vi "UI.vi"() -> ()   [LabVIEW 2020]
panel:
  out "elements":dbl[](array[numeric])
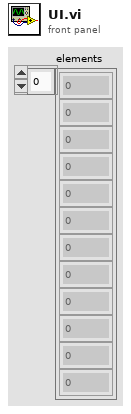
[diagram p1: front panel]
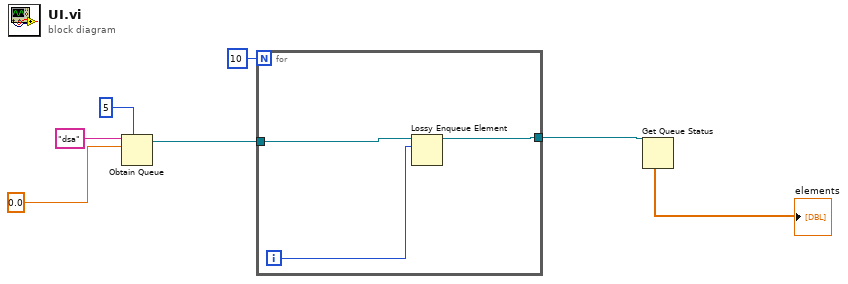
[diagram p0: block diagram]
diagram:
  n1 = Obtain Queue(max queue size (-1, unlimited)=5, name (unnamed)="dsa", element data type=0.0) -> (queue out=w3:refnum<queue>)  [unwired: 2 in, 2 out]
  n2 = for {
    N: 10 -> [_]
    tunnel: w3 -> [w10]
    tunnel: [w8] -> w1
    i -> [w9]
    n3 = Lossy Enqueue Element(queue=w10, element=w9) -> (queue out=w8:refnum<queue>)  [unwired: 1 in, 3 out]
  }
  n4 = Get Queue Status(queue=w1) -> (elements=→"elements":dbl[])  [unwired: 2 in, 7 out]
